vi "SimpleGCLabview.vi"() -> ()   [LabVIEW 2018]
uses:
  <vilib>/Enthought/Python Integration Toolkit/api/Unpack Double.vi
  <vilib>/Enthought/Python Integration Toolkit/Python Integration Toolkit.lvlib
panel:
  out "Function name":string
  out "CH4 mol fraction 3":dbl
  out "O2 mol fraction 2":dbl
  out "CO2 mol fraction":dbl
  in  "Numeric":dbl
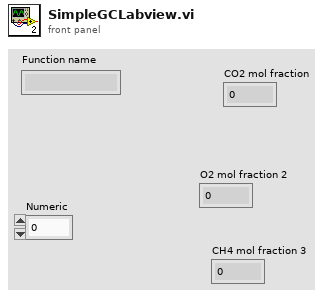
[diagram p1: front panel]
types:
  T1 = typedef "Python Integration Toolkit.lvlib/Session ID.ctl" = u64
  T2 = typedef "Python Integration Toolkit.lvlib/Python Objects.ctl" = variant
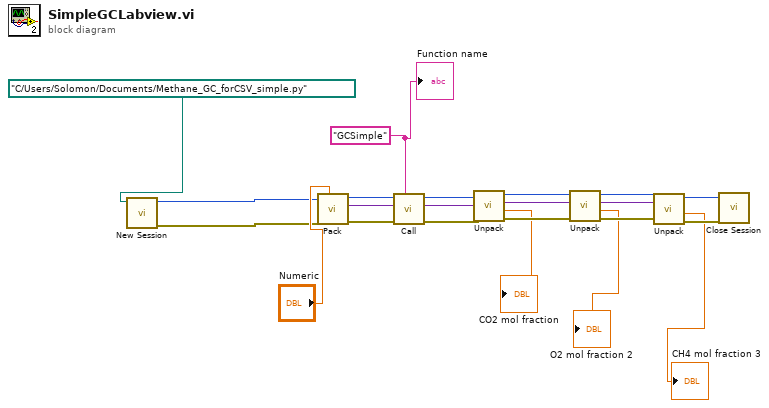
[diagram p0: block diagram]
diagram:
  w3 = "GCSimple" ("Function Name")
  n1 = call <vilib>:"New Session.vi"("Path to Python Module (.py File)"=path "C:/Users/Solomon/Documents/Methane_GC_forCSV_simple.py") -> ("error out"=w1:errorcluster, "Session ID out"=w2:T1)  [unwired: 9 in]
  n2 = call <vilib>:"Pack.vi"("Argument"="Numeric", "error in (no error)"=w1, "Session ID"=w2) -> ("error out"=w19:errorcluster, "Python Object References Out"=w8:T2, "Session ID out"=w20:T1)  [unwired: 6 in]
  n3 = call <vilib>:"Call.vi"("Function or Method Name"=w3, "error in (no error)"=w19, "Python Object References In"=w8, "Session ID"=w20) -> ("error out"=w14:errorcluster, "Python Object References Out"=w7:T2, "Session ID out"=w17:T1)  [unwired: 5 in]
  n4 = call-poly <vilib>:"Unpack.vi"("error in (no error)"=w14, "Python Object References In"=w7, "Session ID"=w17) -> ("error out"=w13:errorcluster, "Value"=→"CO2 mol fraction":dbl, "Python Object References Out"=w6:T2, "Session ID out"=w16:T1)  [unwired: 5 in]
  n5 = call-poly <vilib>:"Unpack.vi"("error in (no error)"=w13, "Python Object References In"=w6, "Session ID"=w16) -> ("error out"=w12:errorcluster, "Value"=→"O2 mol fraction 2":dbl, "Python Object References Out"=w5:T2, "Session ID out"=w15:T1)  [unwired: 5 in]
  n6 = call-poly <vilib>:"Unpack.vi"("error in (no error)"=w12, "Python Object References In"=w5, "Session ID"=w15) -> ("error out"=w21:errorcluster, "Value"=→"CH4 mol fraction 3":dbl, "Session ID out"=w22:T1)  [unwired: 5 in, 1 out]
  n7 = call <vilib>:"Close Session.vi"("error in (no error)"=w21, "Session ID"=w22) -> ()  [unwired: 9 in, 1 out]
  "Function name" <- w3
